vi "呈现图片.vi"(8 "error in (no error)":errorcluster caption="错误输入（无错误）", 11 "图形 输入":refnum<class "图形.lvclass"> caption="DNL_LabVIEW Object in") -> (0 "error out":errorcluster caption="错误输出", 2 "Picture":picture caption="图片", 3 "图形 输出":refnum<class "图形.lvclass"> caption="DNL_LabVIEW Object out")   [LabVIEW 2011, in "图形.lvclass"]
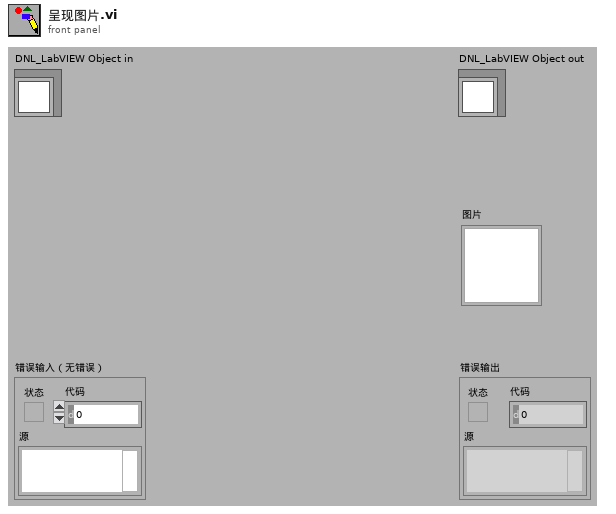
[diagram p1: front panel]
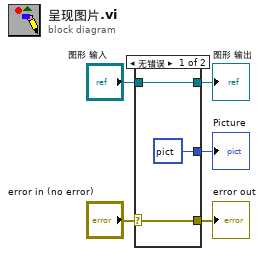
[diagram p0: block diagram]
diagram:
  n1 = case shown="无错误" "error in (no error)" {
    selector: "error in (no error)" -> [w7 w10]
    tunnel: [w7 w10] -> w4
    tunnel: [w8 w9] -> w2
    tunnel: "图形 输入" -> [w8 w9]
    tunnel: [picture data[5B] ("Picture") _] -> w1
    frame No Error {
    }
    frame Error {
    }
  }
  "error out" <- w4
  "图形 输出" <- w2
  "Picture" <- w1
